vi "Teleop.vi"(10 "Match Info":T1={"Autonomous Elapsed Seconds"=0.0, "TeleOp Elapsed Seconds"=0.0, "Disabled Elapsed Seconds"=0.0, "Visited Autonomous"=FALSE, "Visited TeleOp"=FALSE, "Visited Disabled"=FALSE, "Autonomous Settings"={"Autonomous Style"=enum."Independent", "VI Refnum"=refnum}}, 11 "Call Context":T2) -> ()   [LabVIEW 2016]
doc: "This VI is called for each TeleOp packet received from the DS where the robot is not disabled. It is often used to read from the joysticks and update I/O or to update setpoints for timed control loops. It should complete and return within 20 milliseconds or it may miss DS packets."
uses:
  <vilib>/Rock Robotics/WPI/DriverStation/WPI_DriverStationDerivedRobotMode.ctl
  <vilib>/Rock Robotics/WPI/DriverStation/WPI_DriverStationMatch Info.ctl
  <vilib>/Rock Robotics/WPI/Utilities/WPI_GetSetVariantRefNum.vi
  variables/teleopVars.vi
  <vilib>/Rock Robotics/WPI/Solenoid/Deprecated/WPI_SolenoidSetBool.vi
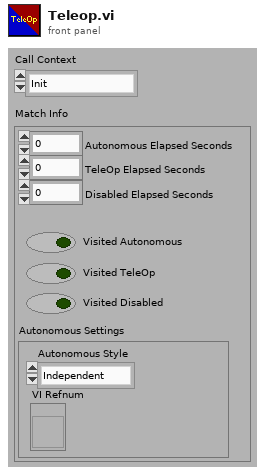
[diagram p1: front panel]
types:
  T1 = typedef "WPI_DriverStationMatch Info.ctl" = cluster{"Autonomous Elapsed Seconds":dbl, "TeleOp Elapsed Seconds":dbl, "Disabled Elapsed Seconds":dbl, "Visited Autonomous":bool, "Visited TeleOp":bool, "Visited Disabled":bool, "Autonomous Settings":cluster{"Autonomous Style":enum16{"Iterative", "Independent"}, "VI Refnum":refnum<vi>}}
  T2 = typedef "WPI_DriverStationDerivedRobotMode.ctl" = enum16{"Init", "Execute", "Stop"}
  T3 = typedef "WPI_SolenoidDevRef.ctl" = cluster{"DevStatus":errorcluster, "Pneumatics Control Module":u8, "Forward Solenoid Channel":T4, "Reverse Solenoid Channel":T4}
  T4 = typedef "WPI_SolenoidChannel.ctl" = enum8{"Solenoid 0", "Solenoid 1", "Solenoid 2", "Solenoid 3", "Solenoid 4", "Solenoid 5", "Solenoid 6", "Solenoid 7", "Invalid"}
  T5 = typedef "WPI_MotorControlDeviceRef.ctl" = cluster{"DeviceStatus":errorcluster, "Type":T6, "PWM":cluster{"PWM Channel":T7, "DeadBand":T8}, "CAN":cluster{"Device Number":u8, "SetOutput VI Ref":variant, "GetOutput VI Ref":variant, "Enable VI Ref":variant, "Disable VI Ref":variant, "Data":variant}, "Invert":bool}
  T6 = typedef "WPI_MotorControlType.ctl" = enum16{"PWM", "CAN"}
  T7 = typedef "FPGA_DIOPWMChannel.ctl" = enum8{"PWM 0", "PWM 1", "PWM 2", "PWM 3", "PWM 4", "PWM 5", "PWM 6", "PWM 7", "PWM 8", "PWM 9", "PWM MXP 0", "PWM MXP 1", "PWM MXP 2", "PWM MXP 3", "PWM MXP 4", "PWM MXP 5", "PWM MXP 6", "PWM MXP 7", "PWM MXP 8", "PWM MXP 9", "Invalid"}
  T8 = typedef "WPI_PWMDeadband.ctl" = cluster{"Name":string, "maxPositivePwm":i32, "minPositivePwm":i32, "centerPwm":i32, "maxNegativePwm":i32, "minNegativePwm":i32, "angularRange":u16}
  T9 = typedef "WPI_RobotDriveDevRef.ctl" = cluster{"DevStatus":errorcluster, "Motors[]":T5[], "Square Inputs":bool, "Max Output":dbl}
  T10 = typedef "WPI_JoystickDevRef.ctl" = cluster{"Device":T11}
  T11 = typedef "WPI_JoystickDeviceEnum.ctl" = enum16{"USB 0", "USB 1", "USB 2", "USB 3", "USB 4", "USB 5"}
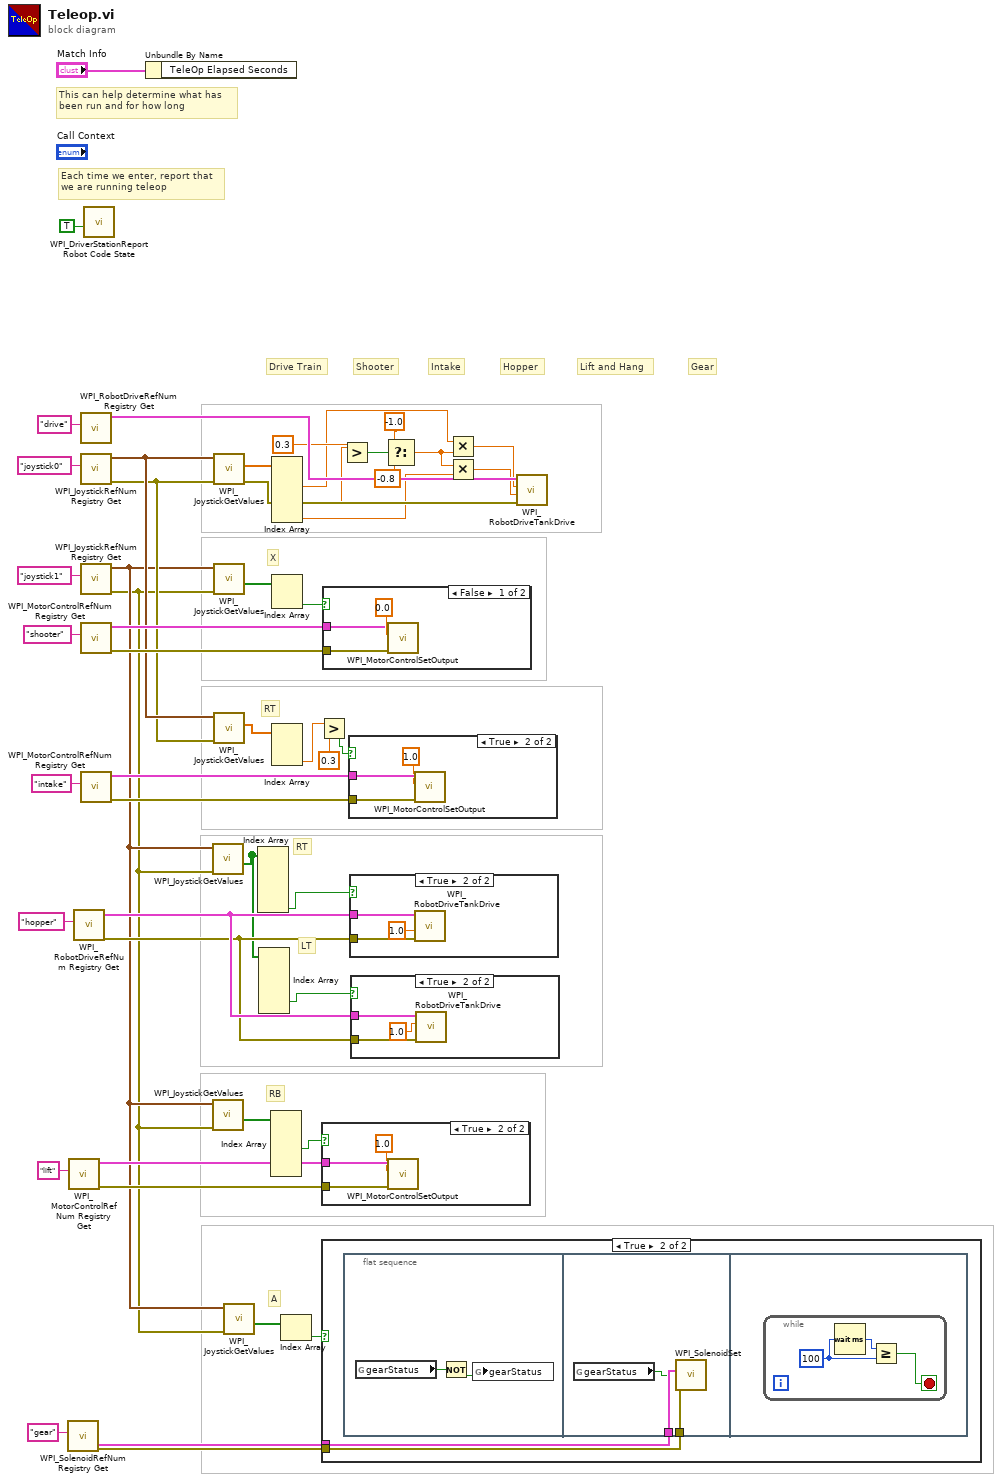
[diagram p0: block diagram]
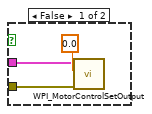
[diagram p3: hidden frame]
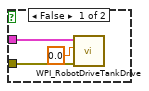
[diagram p4: hidden frame]
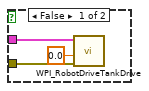
[diagram p5: hidden frame]
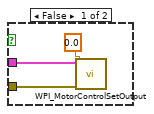
[diagram p6: hidden frame]
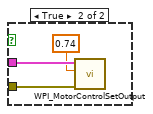
[diagram p7: hidden frame]
diagram:
  # "Gear"
  # "A"
  # "Lift and Hang"
  # "RB"
  # "LT"
  # "RT"
  # "RT"
  # "X"
  # "Hopper"
  # "Intake"
  # "Shooter"
  # "Drive Train"
  # "Each time we enter, report that\nwe are running teleop"
  # "This can help determine what has\nbeen run and for how long"
  n1 = call <vilib>:"WPI_SolenoidRefNum Registry Get.vi"("refnum name"="gear") -> ("error out"=w21:errorcluster, "SolenoidDevRef"=w22:T3)  [unwired: 9 in]
  n2 = call <vilib>:"WPI_MotorControlRefNum Registry Get.vi"("refnum name"="lift") -> ("error out"=w23:errorcluster, "MotorControlDevRef"=w24:T5)  [unwired: 9 in]
  n3 = call <vilib>:"WPI_RobotDriveRefNum Registry Get.vi"("refnum name"="hopper") -> ("error out"=w32:errorcluster, "RobotDriveDevRef"=w33:T9)  [unwired: 9 in]
  n4 = call <vilib>:"WPI_RobotDriveRefNum Registry Get.vi"("refnum name"="drive") -> ("RobotDriveDevRef"=w45:T9)  [unwired: 9 in, 1 out]
  n5 = call <vilib>:"WPI_JoystickRefNum Registry Get.vi"("refnum name"="joystick0") -> ("error out"=w27:errorcluster, "JoystickDevRef"=w28:T10)  [unwired: 9 in]
  n6 = call <vilib>:"WPI_JoystickRefNum Registry Get.vi"("refnum name"="joystick1") -> ("error out"=w16:errorcluster, "JoystickDevRef"=w17:T10)  [unwired: 9 in]
  n7 = call <vilib>:"WPI_MotorControlRefNum Registry Get.vi"("refnum name"="shooter") -> ("error out"=w39:errorcluster, "MotorControlDevRef"=w40:T5)  [unwired: 9 in]
  n8 = call <vilib>:"WPI_MotorControlRefNum Registry Get.vi"("refnum name"="intake") -> ("error out"=w35:errorcluster, "MotorControlDevRef"=w36:T5)  [unwired: 9 in]
  n9 = call <vilib>:"WPI_DriverStationReport Robot Code State.vi"("TeleOp"=TRUE ("Autonomous")) -> ()  [unwired: 10 in, 1 out]
  n10 = Unbundle By Name("Match Info") -> ()  [unwired: 1 out]
  n11 = call <vilib>:"WPI_JoystickGetValues.vi"("error in (no error)"=w16, "JoystickDevRef"=w17) -> ("Buttons"=w1:bool[])  [unwired: 5 in, 4 out]
  n12 = call <vilib>:"WPI_JoystickGetValues.vi"("error in (no error)"=w16, "JoystickDevRef"=w17) -> ("Buttons"=w26:bool[])  [unwired: 5 in, 4 out]
  n13 = call <vilib>:"WPI_JoystickGetValues.vi"("error in (no error)"=w27, "JoystickDevRef"=w28) -> ("error out"=w38:errorcluster, "Axes"=w47:dbl[])  [unwired: 5 in, 3 out]
  n14 = call <vilib>:"WPI_JoystickGetValues.vi"("error in (no error)"=w16, "JoystickDevRef"=w17) -> ("Buttons"=w44:bool[])  [unwired: 5 in, 4 out]
  n15 = call <vilib>:"WPI_JoystickGetValues.vi"("error in (no error)"=w27, "JoystickDevRef"=w28) -> ("Axes"=w31:dbl[])  [unwired: 5 in, 4 out]
  n16 = call <vilib>:"WPI_JoystickGetValues.vi"("error in (no error)"=w16, "JoystickDevRef"=w17) -> ("Buttons"=w19:bool[])  [unwired: 5 in, 4 out]
  n17 = Index Array(array=w1) -> (element #6=w4:bool)  [unwired: 6 in, 5 out]
  n18 = Index Array(array=w1) -> (element #5=w3:bool)  [unwired: 6 in, 5 out]
  n19 = Index Array(array=w26) -> (element #3=w2:bool)  [unwired: 6 in, 5 out]
  n20 = Index Array(array=w47) -> (element #2=w10:dbl, element #4=w15:dbl, element #6=w9:dbl)  [unwired: 6 in, 3 out]
  n21 = Index Array(array=w44) -> (element #2=w43:bool)  [unwired: 2 in, 1 out]
  n22 = Index Array(array=w31) -> (element #3=w5:dbl)  [unwired: 3 in, 2 out]
  n23 = Index Array(array=w19) -> (element=w18:bool)  [unwired: 1 in]
  n24 = Greater?(x=w5, y=0.3) -> (0:w29:bool)
  n25 = case shown="True" w2 {
    tunnel: w24 -> [w52 w56]
    tunnel: w23 -> [w51 w55]
    frame False {
      n26 = call <vilib>:"WPI_MotorControlSetOutput.vi"("error in (no error)"=w51, "Output"=0.0, "MotorControlDevRef"=w52) -> ()  [unwired: 6 in, 3 out]
    }
    frame True {
      n27 = call <vilib>:"WPI_MotorControlSetOutput.vi"("error in (no error)"=w55, "Output"=1.0, "MotorControlDevRef"=w56) -> ()  [unwired: 6 in, 3 out]
    }
  }
  n28 = case shown="True" w18 {
    tunnel: w22 -> [_ w58]
    tunnel: w21 -> [_ w57]
    frame False {
    }
    frame True {
      n29 = flat-sequence {
        tunnel: w58 -> [w63]
        tunnel: w57 -> [w62]
        frame #0 {
          n30 = global read "teleopVars.vi" "gearStatus"() -> (w60:bool)
          n31 = Not(x=w60) -> (.not. x?=w59:bool)
          n32 = global write "teleopVars.vi" "gearStatus"(w59) -> ()
        }
        frame #1 {
          n33 = global read "teleopVars.vi" "gearStatus"() -> (w61:bool)
          n34 = call-poly <vilib>:"WPI_SolenoidSet.vi"("error in (no error)"=w62, "Value"=w61, "SolenoidDevRef"=w63) -> ()  [unwired: 7 in, 2 out]
        }
        frame #2 {
          n35 = while {
            stop <- w64 stop-if-true
            w66 = u32 100 ("milliseconds to wait")
            n36 = Wait (ms)(milliseconds to wait=w66) -> (millisecond timer value=w65:u32)
            n37 = Greater Or Equal?(x=w65, y=w66) -> (x >= y?=w64:bool)
          }
        }
      }
    }
  }
  n38 = case shown="False" w43 {
    tunnel: w40 -> [w68 w72]
    tunnel: w39 -> [w67 w71]
    frame False {
      n39 = call <vilib>:"WPI_MotorControlSetOutput.vi"("error in (no error)"=w67, "Output"=0.0, "MotorControlDevRef"=w68) -> ()  [unwired: 6 in, 3 out]
    }
    frame True {
      n40 = call <vilib>:"WPI_MotorControlSetOutput.vi"("error in (no error)"=w71, "Output"=0.74, "MotorControlDevRef"=w72) -> ()  [unwired: 6 in, 3 out]
    }
  }
  n41 = Greater?(x=w15, y=0.3) -> (0:w13:bool)
  n42 = case shown="True" w29 {
    tunnel: w36 -> [w73 w78]
    tunnel: w35 -> [w74 w77]
    frame False {
      n43 = call <vilib>:"WPI_MotorControlSetOutput.vi"("error in (no error)"=w74, "Output"=0.0, "MotorControlDevRef"=w73) -> ()  [unwired: 6 in, 3 out]
    }
    frame True {
      n44 = call <vilib>:"WPI_MotorControlSetOutput.vi"("error in (no error)"=w77, "Output"=1.0, "MotorControlDevRef"=w78) -> ()  [unwired: 6 in, 3 out]
    }
  }
  n45 = case shown="True" w4 {
    tunnel: w33 -> [w80 w83]
    tunnel: w32 -> [w81 w84]
    frame False {
      n46 = call <vilib>:"WPI_RobotDriveTankDrive.vi"("error in (no error)"=w81, "Right axis value"=0.0, "RobotDriveDevRef"=w80) -> ()  [unwired: 6 in, 3 out]
    }
    frame True {
      n47 = call <vilib>:"WPI_RobotDriveTankDrive.vi"("error in (no error)"=w84, "Right axis value"=1.0, "RobotDriveDevRef"=w83) -> ()  [unwired: 6 in, 3 out]
    }
  }
  n48 = case shown="True" w3 {
    tunnel: w33 -> [w86 w89]
    tunnel: w32 -> [w87 w90]
    frame False {
      n49 = call <vilib>:"WPI_RobotDriveTankDrive.vi"("error in (no error)"=w87, "Left axis value"=0.0 ("Right axis value"), "RobotDriveDevRef"=w86) -> ()  [unwired: 6 in, 3 out]
    }
    frame True {
      n50 = call <vilib>:"WPI_RobotDriveTankDrive.vi"("error in (no error)"=w90, "Left axis value"=1.0 ("Right axis value"), "RobotDriveDevRef"=w89) -> ()  [unwired: 6 in, 3 out]
    }
  }
  n51 = Select(t=-1.0, s=w13, f=-0.8) -> (s? t:f=w8:dbl)
  n52 = Multiply(x=w10, y=w8) -> (x*y=w6:dbl)
  n53 = Multiply(x=w8, y=w9) -> (x*y=w7:dbl)
  n54 = call <vilib>:"WPI_RobotDriveTankDrive.vi"("error in (no error)"=w38, "Right axis value"=w7, "Left axis value"=w6, "RobotDriveDevRef"=w45) -> ()  [unwired: 5 in, 3 out]
